vi "Module Remove.vi"(8 "error in (no error)":errorcluster, 11 "ID":i32) -> (0 "error out":errorcluster, 3 "Module":T1)   [LabVIEW 2022 SP3, in "Core.lvlib"]
uses:
  Core.lvlib
  Controls/Module.ctl
  Controls/Module Instance.ctl
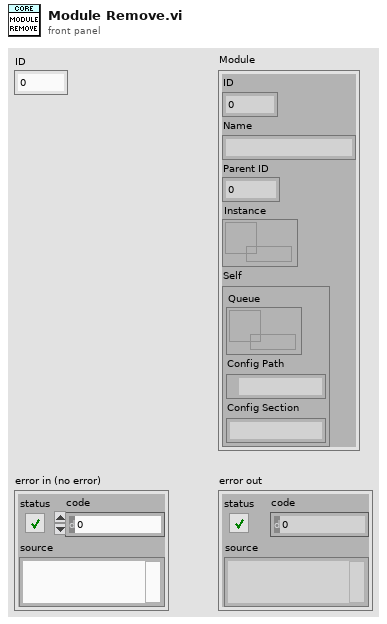
[diagram p1: front panel]
types:
  T1 = typedef "Core.lvlib/Module.ctl" = cluster{"ID":i32, "Name":string, "Parent ID":i32, "Instance":refnum<data-value>, "Self":T2}
  T2 = typedef "Core.lvlib/Module Instance.ctl" = cluster{"Queue":refnum<queue>, "Config Path":path, "Config Section":string}
  T3 = cluster{"ID":i32, "Name":string, "Parent ID":i32, "Instance":refnum<data-value>}[]
  T4 = cluster{"ID":i32, "Name":string, "Parent ID":i32, "Instance":refnum<data-value>}
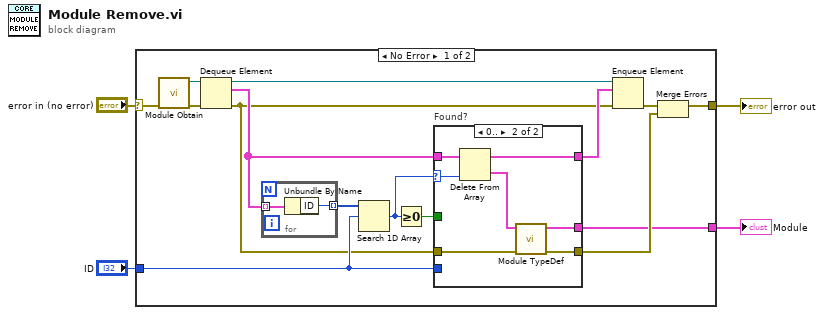
[diagram p0: block diagram]
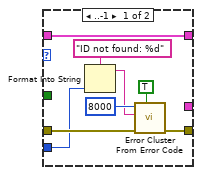
[diagram p2: hidden frame]
diagram:
  n1 = case shown="No Error" "error in (no error)" {
    selector: "error in (no error)" -> [w19 w37]
    tunnel: "ID" -> [w10 _]
    tunnel: [w8 w37] -> w2
    tunnel: [w13 _] -> w1
    frame No Error {
      n2 = call "Module Obtain.vi"("error in (no error)"=w19) -> ("error out"=w18:errorcluster, "Modules"=w17:refnum<queue>)  [unwired: 9 in]
      n3 = Dequeue Element(queue=w17, error in (no error)=w18) -> (queue out=w9:refnum<queue>, element=w15:T3, error out=w5:errorcluster)  [unwired: 1 in, 1 out]
      n4 = for {
        tunnel: w15 -> [w36] mode=indexing
        tunnel: [w35] -> w16 mode=indexing
        n5 = Unbundle By Name(w36) -> ("ID"=w35:i32)
      }
      n6 = Search 1D Array(1D array=w16, element=w10) -> (index of element=w12:i32)  [unwired: 1 in]
      n7 = Greater Or Equal To 0?(x=w12) -> (x >= 0?=w11:bool)
      n8 = case "Found?" shown="0.." w12 {
        selector: w12 -> [_ w29]
        tunnel: w15 -> [w20 w34]
        tunnel: w5 -> [w27 w33]
        tunnel: [w26 w32] -> w14
        tunnel: [_ w30] -> w13
        tunnel: w11 -> [_ _]
        tunnel: w10 -> [w23 _]
        tunnel: [w20 w28] -> w6
        frame ..-1 {
          n9 = Format Into String(format string="ID not found: %d", w23) -> (resulting string=w21:string)  [unwired: 2 in, 1 out]
          n10 = call <vilib>:"Error Cluster From Error Code.vi"("show call chain? (False)"=TRUE, "error in (no error)"=w27, "error message (\"\")"=w21, "error code (0)"=8000) -> ("error out"=w26:errorcluster)  [unwired: 5 in]
        }
        frame 0.. {
          n11 = Delete From Array(array=w34, index=w29) -> (deleted portion=w31:T4, array with subset deleted=w28:T3)  [unwired: 1 in]
          n12 = call "Module TypeDef.vi"("error in (no error)"=w33, "Module in"=w31) -> ("error out"=w32:errorcluster, "Module"=w30:T1)  [unwired: 8 in]
        }
      }
      n13 = Enqueue Element(queue=w9, element=w6, error in (no error)=w5) -> (error out=w7:errorcluster)  [unwired: 1 in, 2 out]
      n14 = Merge Errors(w7, w14) -> (w8:errorcluster)
    }
    frame Error {
    }
  }
  "error out" <- w2
  "Module" <- w1
